vi "ALR redefine.vi"(4 "ALRParamTable":string="f_alr_3", 6 "conninfo":T4={"host"="localhost", "port"="5432", "client_encoding"="WIN1251", "dbname"="data", "user"="postgres", "password"=""}, 8 "error in (no error)":errorcluster, 9 "LevelTable":string[](array[string]), 10 "fcodealr_full":string[](array[string]), 11 "Alarms in":T1) -> (0 "error":errorcluster, 3 "Alarms out":T1)   [LabVIEW 2019, in "Alarms.lvlib"]
uses:
  Alarms.lvlib
  Database/ctl/Coninfo.ctl
  Ctl/Alarms.ctl
  Ctl/ALR_defs.ctl
  Ctl/ALRs_State.ctl
  Ctl/ALR_ON_OFF.ctl
  Ctl/ALR_Parameters.ctl
  Ctl/ALR code.ctl
  Ctl/ALR type.ctl
  Database/select_initial_alr.vi
  Database/PostgreSQL2LabVIEW/libpqUtility/src/PQclose.vi
  Database/PostgreSQL2LabVIEW/libpqUtility/src/PQconnect.vi
  Database/PostgreSQL2LabVIEW/libpqlv/src/PQfinish.vi
  Database/PostgreSQL2LabVIEW/libpqlv/src/PQconnectdb.vi
  Database/PostgreSQL2LabVIEW/libpqlv/src/PQerrorMessage.vi
  Database/PostgreSQL2LabVIEW/libpqlv/src/PQstatus.vi
  <vilib>/dlg_ctls.llb/Space Constant.vi
  <userlib>/_OpenG.lib/lvdata/lvdata.llb/Get Strings from Enum__ogtk.vi
  Database/PostgreSQL2LabVIEW/libpqUtility/src/PQgetTable.vi
  Database/Progress.vi
  Database/PostgreSQL.lvlib
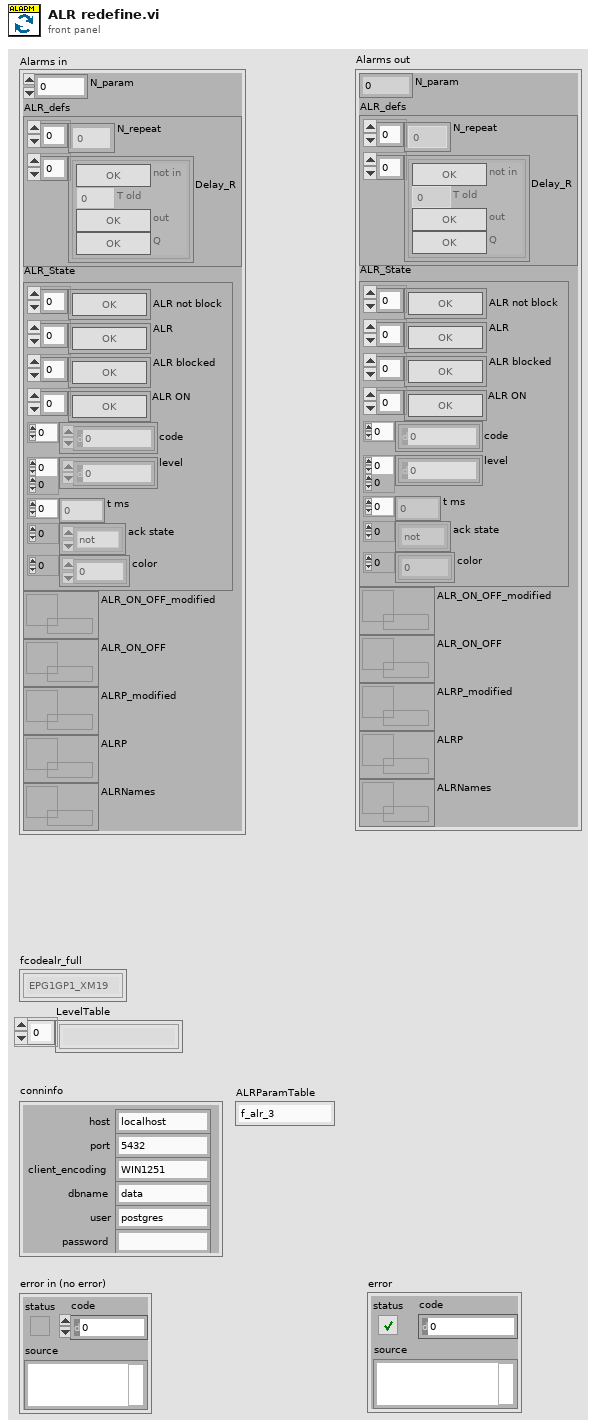
[diagram p1: front panel]
types:
  T1 = typedef "Alarms.lvlib/Alarms.ctl" = cluster{"N_param":i32, "ALR_defs":T2, "ALR_State":T3, "ALR_ON_OFF_modified":refnum<data-value>, "ALR_ON_OFF":refnum<data-value>, "ALRP_modified":refnum<data-value>, "ALRP":refnum<data-value>, "ALRNames":refnum<data-value>}
  T2 = typedef "Alarms.lvlib/ALR_defs.ctl" = cluster{"N_repeat":u32[], "Delay_R":cluster{"not in":bool, "T old":u32, "out":bool, "Q":bool}[]}
  T3 = typedef "Alarms.lvlib/ALRs_State.ctl" = cluster{"ALR not block":bool[], "ALR":bool[], "ALR blocked":bool[], "ALR ON":bool[], "code":i32[], "level":i32[][], "t ms":u32[], "ack state":enum32{"not", "tripped", "reset", "ack"}[], "color":u32[]}
  T4 = typedef "PostgreSQL.lvlib/Coninfo.ctl" = cluster{"host":string, "port":string, "client_encoding":string, "dbname":string, "user":string, "password":string}
  T5 = typedef "Alarms.lvlib/ALR_Parameters.ctl" = cluster{"ALR code":T6[], "ALR type":T7[], "ALRParam":u32[][]}
  T6 = typedef "Alarms.lvlib/ALR code.ctl" = enum16{"CONN", "H", "HH", "L", "LL", "SERR", "ON", "OFF", "XM19", "XM24", "XM47", "XM51", "XM52", "XM53", "XM54", "XM55", "XM56", "XM61", "XM62", "XM63", "XM64", "XM65", "XM66"}
  T7 = typedef "Alarms.lvlib/ALR type.ctl" = enum16{"ACD", "ACDR", "ALRN", "ALR"}
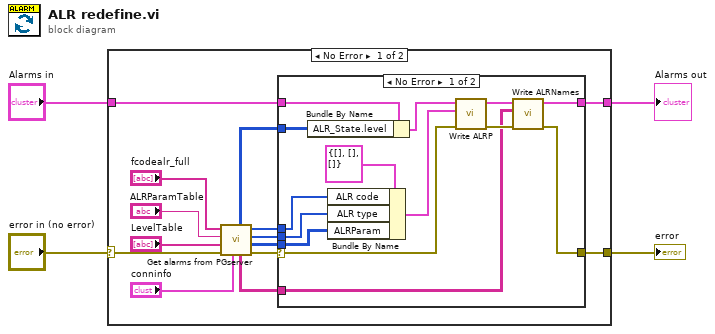
[diagram p0: block diagram]
diagram:
  n1 = case shown="No Error" "error in (no error)" {
    selector: "error in (no error)" -> [w10 w36]
    tunnel: [w8 w36] -> w4
    tunnel: "Alarms in" -> [w9 w35]
    tunnel: [w7 w35] -> w3
    frame No Error {
      n2 = call "Get alarms from PGserver.vi"("conninfo"="conninfo", "error in"=w10, "LevelTable"="LevelTable", "ALRParamTable"="ALRParamTable", "fcodealr_full"="fcodealr_full") -> ("error out"=w15:errorcluster, "ALRParameters table"=w11:u32[][], "ALR type"=w18:T7[], "ALR code"=w16:T6[], "ALRNames"=w17:string[][], "ALRLevel table"=w6:i32[][])  [unwired: 1 in]
      n3 = case shown="No Error" w15 {
        selector: w15 -> [w19 w33]
        tunnel: w11 -> [w27 _]
        tunnel: w16 -> [w29 _]
        tunnel: w17 -> [w20 _]
        tunnel: w18 -> [w28 _]
        tunnel: [w22 w33] -> w8
        tunnel: w9 -> [w31 w34]
        tunnel: [w24 w34] -> w7
        tunnel: w6 -> [w32 _]
        frame No Error {
          n4 = Bundle By Name(cluster=w31, "ALR_State.level"=w32) -> (w26:T1)
          n5 = Bundle By Name(cluster=T5 {"ALR code"=[], "ALR type"=[], "ALRParam"=[]} ("data value"), "ALR code"=w29, "ALR type"=w28, "ALRParam"=w27) -> (w21:T5)
          n6 = call "Write ALRP.vi"("error in (no error)"=w19, "ALRP"=w21, "Alarms in"=w26) -> ("error out"=w23:errorcluster, "Alarms out"=w25:T1)  [unwired: 7 in]
          n7 = call "Write ALRNames.vi"("error in (no error)"=w23, "ALRNames"=w20, "Alarms in"=w25) -> ("error out"=w22:errorcluster, "Alarms out"=w24:T1)  [unwired: 7 in]
        }
        frame Error {
        }
      }
    }
    frame Error {
    }
  }
  "error" <- w4
  "Alarms out" <- w3
